vi "setPhaseBlazingTable.vi"(2 "-¹..¹ range control":enum16{"wrap round", "cast to range"}(ring)=enum."cast to range", 3 "Anchor Points":cluster{"X":dbl, "Y":dbl}[](array[cluster]), 4 "#elements (default 256)":i32=32) -> (0 "blazing graph":cluster{dbl, dbl}[](graph), 1 "blazing table":dbl[](array[numeric])=[3.0, 0.0, 0.0, 0.0, 0.0, 0.0, 0.0, 0.0, 0.0, 0.0, 0.0, 0.0, 0.0, 0.0, 0.0, 0.0, 0.0, 0.0, 0.0, 0.0, 0.0, 0.0, 0.0, 0.0, 0.0, 0.0, 0.0, 0.0, 0.0, 0.0, 0.0, 0.0, 0.0, 0.0, 0.0, 0.0, 0.0, 0.0, 0.0, 0.0, 0.0, 0.0, 0.0, 0.0, 0.0, 0.0, 0.0, 0.0, 0.0, 0.0, 0.0, 0.0, 0.0, 0.0, 0.0, 0.0, 0.0, 0.0, 0.0, 0.0, 0.0, 0.0, 0.0, 0.0, 0.0, 0.0, 0.0, 0.0, 0.0, 0.0, 0.0, 0.0, 0.0, 0.0, 0.0, 0.0, 0.0, 0.0, 0.0, 0.0, 0.0, 0.0, 0.0, 0.0, 0.0, 0.0, 0.0, 0.0, 0.0, 0.0, 0.0, 0.0, 0.0, 0.0, 0.0, 0.0, 0.0, 0.0, 0.0, 0.0, 0.0, 0.0, 0.0, 0.0, 0.0, 0.0, 0.0, 0.0, 0.0, 0.0, 0.0, 0.0, 0.0, 0.0, 0.0, 0.0, 0.0, 0.0, 0.0, 0.0, 0.0, 0.0, 0.0, 0.0, 0.0, 0.0, 0.0, 0.0, 0.0, 0.0, 0.0, 0.0, 0.0, 0.0, 0.0, 0.0, 0.0, 0.0, 0.0, 0.0, 0.0, 0.0, 0.0, 0.0, 0.0, 0.0, 0.0, 0.0, 0.0, 1.0, 1.0, 1.0, 1.0, 1.0, 1.0, 1.0, 1.0, 1.0, 1.0, 1.0, 1.0, 1.0, 1.0, 1.0, 1.0, 1.0, 1.0, 1.0, 1.0, 1.0, 1.0, 1.0, 1.0, 1.0, 1.0, 1.0, 1.0, 1.0, 1.0, 1.0, 1.0, 1.0, 1.0, 1.0, 1.0, 1.0, 1.0, 1.0, 1.0, 1.0, 2.0, 2.0, 2.0, 2.0, 2.0, 2.0, 2.0, 2.0, 2.0, 2.0, 2.0, 2.0, 2.0, 2.0, 2.0, 2.0, 2.0, 2.0, 2.0, 2.0, 2.0, 2.0, 2.0, 2.0, 2.0, 2.0, 2.0, 2.0, 2.0, 2.0, 2.0, 2.0, 2.0, 2.0, 2.0, 2.0, 2.0, 2.0, 2.0, 2.0, 3.0, 3.0, 3.0, 3.0, 3.0, 3.0, 3.0, 3.0, 3.0, 3.0, 3.0, 3.0, 3.0, 3.0, 3.0, 3.0, 3.0, 3.0, 3.0, 3.0, 3.0, 3.0, 3.0, 3.0, 3.0, 3.0])   [LabVIEW 2019]
uses:
  <vilib>/Analysis/NI_AALPro.lvlib
panel:
  # "This should have range 0 to 1, with -pi->pi mapped onto the range if its indices for X"
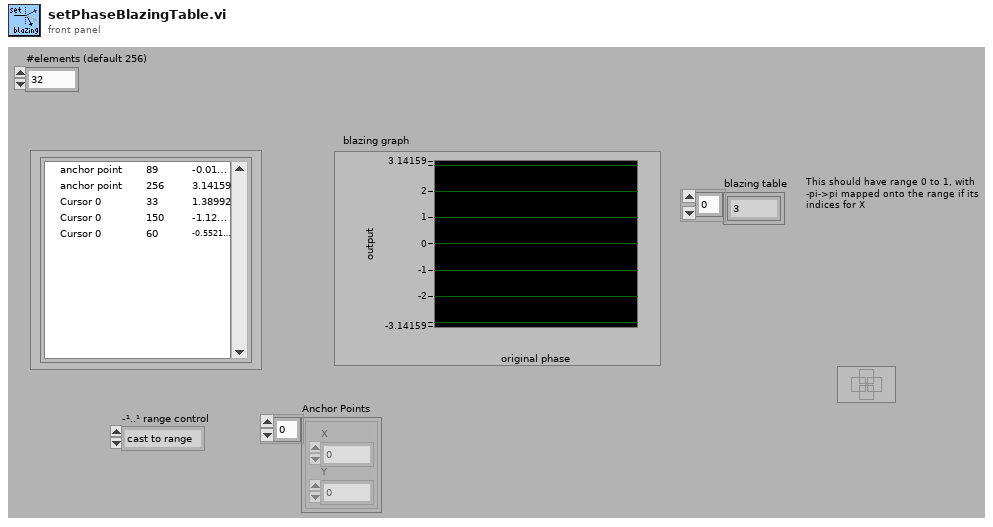
[diagram p1: front panel]
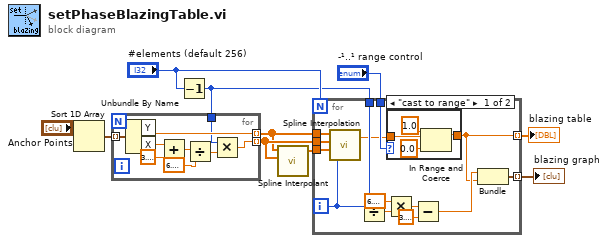
[diagram p0: block diagram]
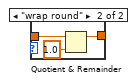
[diagram p2: hidden frame]
diagram:
  n1 = Sort 1D Array(array="Anchor Points") -> (sorted array=w7:cluster{"X":dbl, "Y":dbl}[])
  n2 = Decrement(x="#elements (default 256)") -> (x-1=w4:i32)
  n3 = for {
    tunnel: w7 -> [w19] mode=indexing
    tunnel: [w18] -> w9 mode=indexing
    tunnel: [w12] -> w10 mode=indexing
    tunnel: w4 -> [w11]
    n4 = Unbundle By Name(w19) -> ("Y"=w18:dbl, "X"=w17:dbl)
    n5 = Add(x=w17, y=3.141592653589793) -> (x+y=w15:dbl)
    n6 = Divide(x=w15, y=6.283185307179586) -> (x/y=w13:dbl)
    n7 = Multiply(x=w11, y=w13) -> (x*y=w12:dbl)
  }
  n8 = call <vilib>:"Spline Interpolant.vi"("X"=w10, "Y"=w9) -> ("Interpolant"=w8:dbl[])  [unwired: 2 in, 1 out]
  n9 = for {
    N: "#elements (default 256)" -> [_]
    tunnel: w8 -> [w33]
    tunnel: w9 -> [w32]
    tunnel: w10 -> [w31]
    tunnel: w4 -> [w29]
    tunnel: "-¹..¹ range control" -> [w24]
    tunnel: [w20] -> w2 mode=indexing
    tunnel: [w22] -> w1 mode=indexing
    i -> [w30]
    n10 = call <vilib>:"Spline Interpolation.vi"("x value"=w30, "Interpolant"=w33, "X"=w31, "Y"=w32) -> ("interpolation value"=w23:dbl)  [unwired: 1 out]
    n11 = Divide(x=w30, y=w29) -> (x/y=w28:dbl)
    n12 = Multiply(x=6.283185307179586, y=w28) -> (x*y=w26:dbl)
    n13 = case shown="\"cast to range\"" w24 {
      tunnel: [w34 w38] -> w20
      tunnel: w23 -> [w37 w40]
      frame "cast to range" {
        n14 = In Range and Coerce(upper limit=1.0 ("x"), x=w37, lower limit=0.0 ("x")) -> (coerced(x)=w34:dbl)  [unwired: 1 out]
      }
      frame "wrap round" {
        n15 = Quotient & Remainder(x=w40, y=1.0) -> (x-y*floor(x/y)=w38:dbl)  [unwired: 1 out]
      }
    }
    n16 = Subtract(x=w26, y=3.141592653589793) -> (x-y=w21:dbl)
    n17 = Bundle(w21, "x"=w20) -> (w22:cluster{dbl, "x":dbl})  [unwired: 1 out]
  }
  "blazing graph" <- w1
  "blazing table" <- w2
